vi "Message Handling Loop - Data.vi"(8 "error in":errorcluster, 9 "Message Queues in":T1, 10 "User Event Bundle":T2) -> (0 "error out":errorcluster)   [LabVIEW 2018]
uses:
  Type Defs/User Events.ctl
  Support/Message Queue/All Message Queues.ctl
  Support/Message Queue/Message Cluster.ctl
  Type Defs/Data Loop Data.ctl
  Support/Message Queue/Enqueue Message (Single).vi
  <vilib>/Utility/error.llb/Error Cluster From Error Code.vi
  <vilib>/ErrorRing/Error Ring.xnode
  Support/Message Queue/Message Queue.lvlib
  Support/User Events/User Events.lvlib
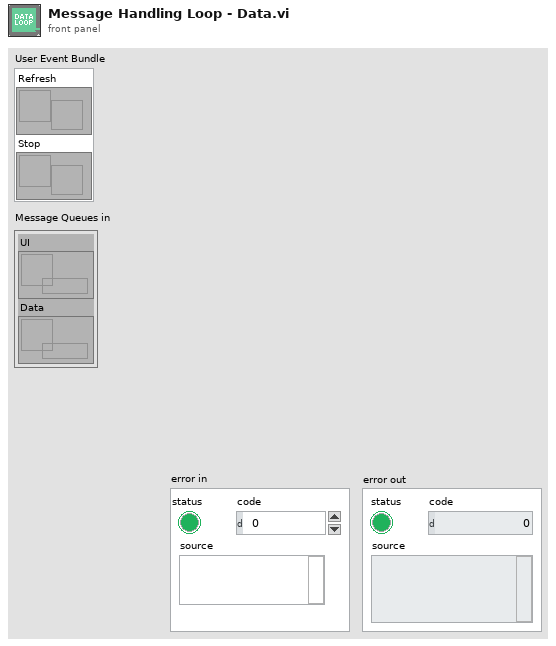
[diagram p1: front panel]
types:
  T1 = typedef "Message Queue.lvlib/All Message Queues.ctl" = cluster{"UI":refnum<queue>, "Data":refnum<queue>}
  T2 = typedef "User Events.ctl" = cluster{"Refresh":refnum<user-event>, "Stop":refnum<user-event>}
  T3 = typedef "Data Loop Data.ctl" = cluster{"Main VI":refnum<vi>, "Update List":i32[], "File Path":path, "Add SR":refnum<vi>, "Remove SR":refnum<vi>, "Refresh SRs":refnum<vi>, "UI":refnum<queue>, "Data":refnum<queue>}
  T4 = typedef "SR Cluster.ctl" = cluster{"Color":u32, "SR Number":i32, "SR Status":T5, "Name":string, "Summary":string, "Last Updated":timestamp, "SR Type":string, "Service Level":string, "Days Open":dbl, "Creation Date":timestamp}
  T5 = typedef "SR Status.ctl" = enum16{"Caller Abandoned", "Created in Error", "Expired", "Forum Resolved AE", "Forum Resolved Customer", "IN WORK", "IN WORK Collab with AES", "IN WORK Collab with PSE", "IN WORK Collab with SE", "IN WORK Customer Added Note", "IN WORK Escalation", "IN WORK Wait on Customer", "Open", "Potentially Resolved", "Presumed Resolved", "RMA Approved for Return", "RMA Closed", "RMA Closed - DOA", "RMA In Progress", "RMA Open", "RMA Waiting on Customer", "Resolved", "Passed Off"}
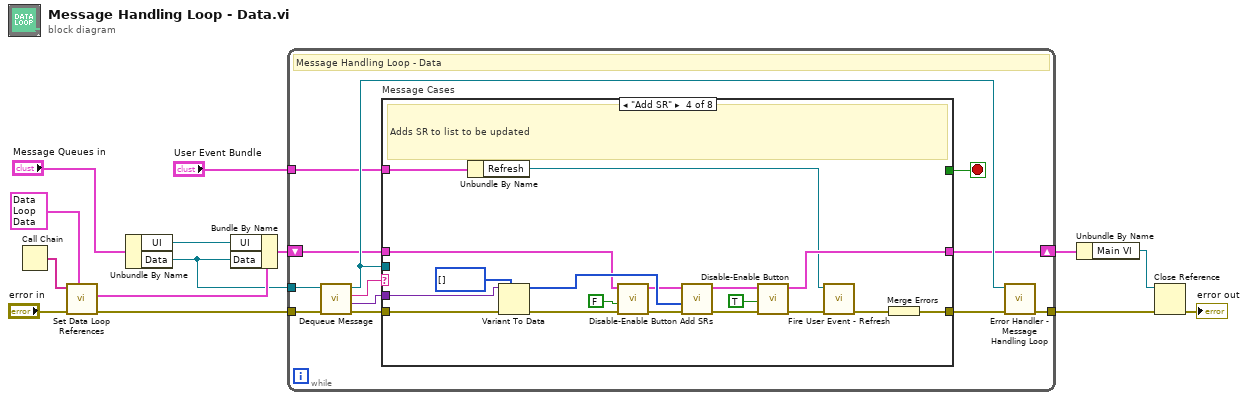
[diagram p0: block diagram]
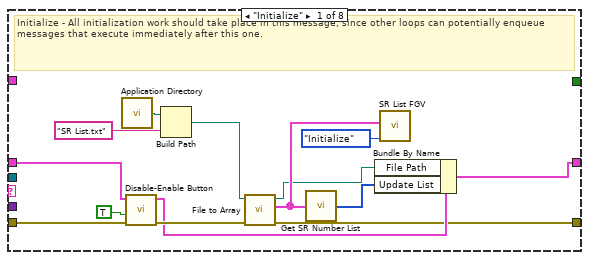
[diagram p2: hidden frame]
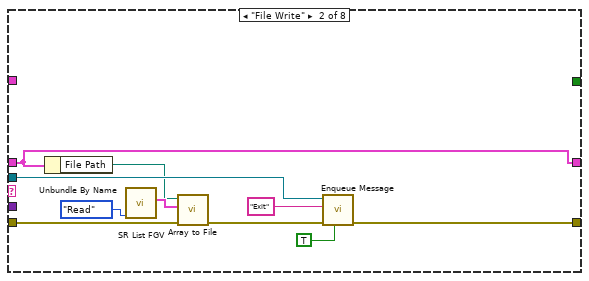
[diagram p3: hidden frame]
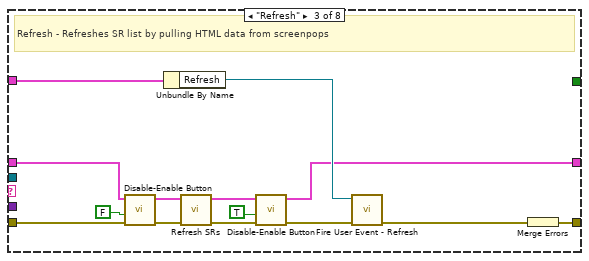
[diagram p4: hidden frame]
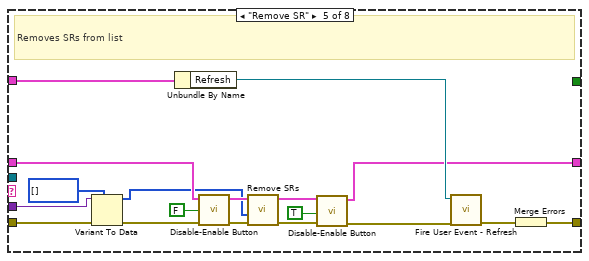
[diagram p5: hidden frame]
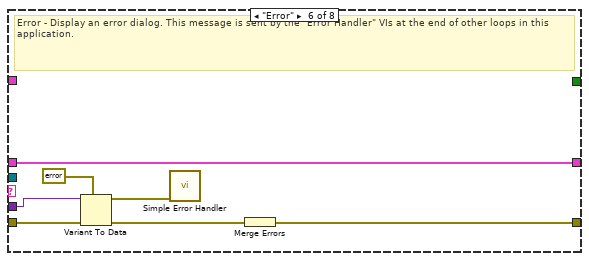
[diagram p6: hidden frame]
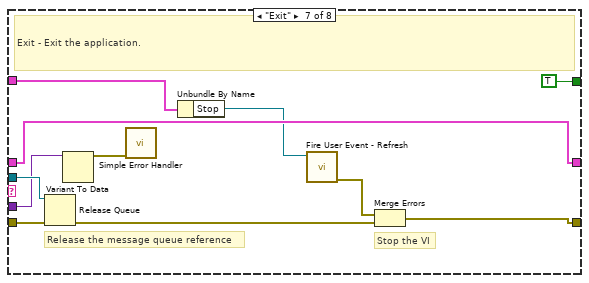
[diagram p7: hidden frame]
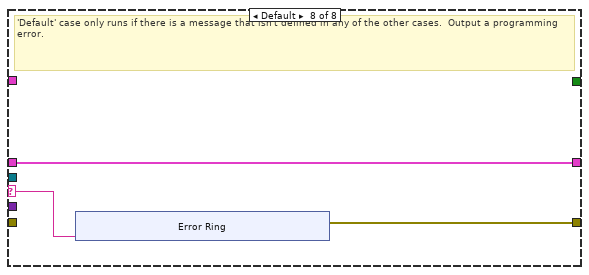
[diagram p8: hidden frame]
diagram:
  n1 = Call Chain() -> (call chain=w13:string[])
  n2 = call "Set Data Loop References.vi"("Data Loop Data in"=T3 {"Main VI"=refnum, "Update List"=[], "File Path"=path "", "Add SR"=refnum, "Remove SR"=refnum, "Refresh SRs"=refnum, "UI"=refnum, "Data"=refnum}, "error in"="error in", "call chain"=w13) -> ("error out"=w9:errorcluster, "Data Loop Data out"=w7:T3)  [unwired: 7 in]
  n3 = Unbundle By Name("Message Queues in") -> ("UI"=w4:refnum<queue>, "Data"=w3:refnum<queue>)
  n4 = Bundle By Name(cluster=w7, "UI"=w4, "Data"=w3) -> (w6:T3)
  n5 = while {
    tunnel: w3 -> [w22]
    tunnel: [w20] -> w11
    shift-right: [w17] -> w2
    shift-left: w6 -> [w18]
    tunnel: w9 -> [w16]
    tunnel: "User Event Bundle" -> [w15]
    stop <- w26 stop-if-true
    # "Message Handling Loop - Data"
    n6 = call "Dequeue Message.vi"("error in (no error)"=w16, "Message Queue"=w22) -> ("error out"=w25:errorcluster, "Message Data"=w23:variant, "Message"=w24:string, "dup Message Queue"=w21:refnum<queue>)  [unwired: 6 in]
    n7 = case "Message Cases" shown="\"Add SR\"" w24 {
      selector: w24 -> [_ _ _ _ _ _ _ w120]
      tunnel: w21 -> [_ w50 _ _ _ _ w118 _]
      tunnel: w25 -> [w30 w45 w51 w79 w97 w107 w114 _]
      tunnel: [w27 w49 w64 w82 w100 w102 w115 w121] -> w19
      tunnel: [_ _ _ _ _ _ TRUE _] -> w26
      tunnel: w23 -> [_ _ _ w81 w99 w106 w112 _]
      tunnel: w18 -> [w31 w42 w52 w70 w91 w101 w111 w119]
      tunnel: [w39 w42 w55 w72 w88 w101 w111 w119] -> w17
      tunnel: w15 -> [_ _ w61 w69 w96 _ w110 _]
      frame "Initialize" {
        # "Initialize - All initialization work should take place in this message, since other loops can potentially enqueue messages that execute immediately after this one."
        n8 = call <vilib>:"Application Directory.vi"() -> ("Application Directory"=w38:path)
        n9 = call "Disable-Enable Button.vi"("error in"=w30, "Enabled?"=TRUE, "Data Loop Data in"=w31) -> ("error out"=w29:errorcluster, "Data Loop Data out"=w28:T3)  [unwired: 7 in]
        n10 = Build Path(base path=w38, name or relative path="SR List.txt") -> (appended path=w36:path)
        n11 = call "File to Array.vi"("error in"=w29, "file path in"=w36) -> ("error out"=w27:errorcluster, "list out"=w35:T4[], "file path out"=w32:path)  [unwired: 7 in]
        n12 = call "Get SR Number List.vi"("list in"=w35) -> ("SR number array out"=w33:i32[])  [unwired: 4 in]
        n13 = Bundle By Name(cluster=w28, "File Path"=w32, "Update List"=w33) -> (w39:T3)
        n14 = call "SR List FGV.vi"("Operation"=enum16{"Initialize", "Write", "Read", "Clear"}."Initialize", "list in"=w35) -> ()  [unwired: 8 in, 2 out]
      }
      frame "File Write" {
        n15 = Unbundle By Name(w42) -> ("File Path"=w41:path)
        n16 = call "SR List FGV.vi"("Operation"=enum16{"Initialize", "Write", "Read", "Clear"}."Read") -> ("list out"=w44:T4[])  [unwired: 9 in, 1 out]
        n17 = call "Array to File.vi"("error in"=w45, "array in"=w44, "file path in"=w41) -> ("error out"=w46:errorcluster)  [unwired: 7 in, 1 out]
        n18 = call-poly "Enqueue Message.vi"("Priority Message? (F)"=TRUE, "error in (no error)"=w46, "Message"="Exit", "Message Queue"=w50) -> ("error out"=w49:errorcluster)  [unwired: 6 in, 1 out]
      }
      frame "Refresh" {
        # "Refresh - Refreshes SR list by pulling HTML data from screenpops"
        n19 = call "Disable-Enable Button.vi"("error in"=w51, "Enabled?"=FALSE, "Data Loop Data in"=w52) -> ("error out"=w63:errorcluster, "Data Loop Data out"=w59:T3)  [unwired: 7 in]
        n20 = Unbundle By Name(w61) -> ("Refresh"=w60:refnum<user-event>)
        n21 = call "Refresh SRs.vi"("error in"=w63, "Data Loop Data in"=w59) -> ("error out"=w56:errorcluster, "Data Loop Data out"=w58:T3)  [unwired: 8 in]
        n22 = call "Disable-Enable Button.vi"("error in"=w56, "Enabled?"=TRUE, "Data Loop Data in"=w58) -> ("error out"=w54:errorcluster, "Data Loop Data out"=w55:T3)  [unwired: 7 in]
        n23 = call "Fire User Event - Refresh.vi"("error in (no error)"=w54, "Refresh"=w60) -> ("error out"=w53:errorcluster)  [unwired: 9 in]
        n24 = Merge Errors(w53) -> (w64:errorcluster)
      }
      frame "Add SR" {
        # "Adds SR to list to be updated"
        n25 = Unbundle By Name(w69) -> ("Refresh"=w68:refnum<user-event>)
        n26 = Variant To Data(error in=w79, type=i32[] [], Variant=w81) -> (data=w76:i32[], error out=w65:errorcluster)
        n27 = call "Disable-Enable Button.vi"("error in"=w65, "Enabled?"=FALSE, "Data Loop Data in"=w70) -> ("error out"=w75:errorcluster, "Data Loop Data out"=w71:T3)  [unwired: 7 in]
        n28 = call "Add SRs.vi"("error in"=w75, "entered SRs in"=w76, "Data Loop Data in"=w71) -> ("error out"=w74:errorcluster, "Data Loop Data out"=w73:T3)  [unwired: 7 in]
        n29 = call "Disable-Enable Button.vi"("error in"=w74, "Enabled?"=TRUE, "Data Loop Data in"=w73) -> ("error out"=w67:errorcluster, "Data Loop Data out"=w72:T3)  [unwired: 7 in]
        n30 = call "Fire User Event - Refresh.vi"("error in (no error)"=w67, "Refresh"=w68) -> ("error out"=w66:errorcluster)  [unwired: 9 in]
        n31 = Merge Errors(w66) -> (w82:errorcluster)
      }
      frame "Remove SR" {
        # "Removes SRs from list"
        n32 = Variant To Data(error in=w97, type=i32[] [], Variant=w99) -> (data=w83:i32[], error out=w84:errorcluster)
        n33 = Unbundle By Name(w96) -> ("Refresh"=w95:refnum<user-event>)
        n34 = call "Disable-Enable Button.vi"("error in"=w84, "Enabled?"=FALSE, "Data Loop Data in"=w91) -> ("error out"=w85:errorcluster, "Data Loop Data out"=w92:T3)  [unwired: 7 in]
        n35 = call "Remove SRs.vi"("error in"=w85, "entered SRs in"=w83, "Data Loop Data in"=w92) -> ("error out"=w87:errorcluster, "Data Loop Data out"=w89:T3)  [unwired: 7 in]
        n36 = call "Disable-Enable Button.vi"("error in"=w87, "Enabled?"=TRUE, "Data Loop Data in"=w89) -> ("error out"=w86:errorcluster, "Data Loop Data out"=w88:T3)  [unwired: 7 in]
        n37 = call "Fire User Event - Refresh.vi"("error in (no error)"=w86, "Refresh"=w95) -> ("error out"=w94:errorcluster)  [unwired: 9 in]
        n38 = Merge Errors(w94) -> (w100:errorcluster)
      }
      frame "Error" {
        # "Error - Display an error dialog. This message is sent by the \"Error Handler\" VIs at the end of other loops in this application."
        n39 = Variant To Data(error in=w107, type=errorcluster {"status"=FALSE, "code"=0, "source"=""} ("error constant"), Variant=w106) -> (data=w104:errorcluster, error out=w103:errorcluster)
        n40 = call <vilib>:"Simple Error Handler.vi"("error in (no error)"=w104) -> ()  [unwired: 4 in, 5 out]
        n41 = Merge Errors(w103) -> (w102:errorcluster)
      }
      frame "Exit" {
        # "Stop the VI"
        # "Release the message queue reference"
        # "Exit - Exit the application."
        n42 = Release Queue(queue=w118, error in (no error)=w114) -> (error out=w116:errorcluster)  [unwired: 1 in, 2 out]
        n43 = Variant To Data(Variant=w112) -> (data=w113:errorcluster)  [unwired: 2 in, 1 out]
        n44 = call <vilib>:"Simple Error Handler.vi"("error in (no error)"=w113) -> ()  [unwired: 4 in, 5 out]
        n45 = Unbundle By Name(w110) -> ("Stop"=w109:refnum<user-event>)
        n46 = call "Fire User Event - Refresh.vi"("Refresh"=w109) -> ("error out"=w108:errorcluster)  [unwired: 10 in]
        n47 = Merge Errors(w108, w116) -> (w115:errorcluster)
      }
      frame Default {
        # "'Default' case only runs if there is a message that isn't defined in any of the other cases.  Output a programming error."
        n48 = xnode "Error Ring"("parameter 0"=w120) -> ("error out"=w121:errorcluster)
      }
    }
    n49 = call "Error Handler - Message Handling Loop.vi"("error in (no error)"=w19, "Message Queue"=w21) -> ("dup error in"=w20:errorcluster)  [unwired: 8 in, 1 out]
  }
  n50 = Unbundle By Name(w2) -> ("Main VI"=w1:refnum<vi>)
  n51 = Close Reference(reference=w1, error in (no error)=w11) -> (error out=→"error out":errorcluster)
